vi "DropDetectionForLinkamForMultipleImages.vi"(6 "Circle Descriptor":cluster{"Min Radius":dbl, "Max Radius":dbl}={"Min Radius"=3.0, "Max Radius"=500.0}, 8 "error in":errorcluster, 9 "Image in":T2(plugin-control), 10 "Minimum match score":dbl=950.0) -> (0 "error out":errorcluster, 1 "Number of matches":i32, 2 "Matches (pixel)":T1(array[cluster]), 3 "Image Out":T2(plugin-control), 4 "Circles (Calibrated)":T3(array[cluster]) {"Position"."Y" format="%.2f"; "Position"."X" format="%.2f"})   [LabVIEW 2013]
uses:
  <vilib>/vision/NI_Vision_Development_Module.lvlib
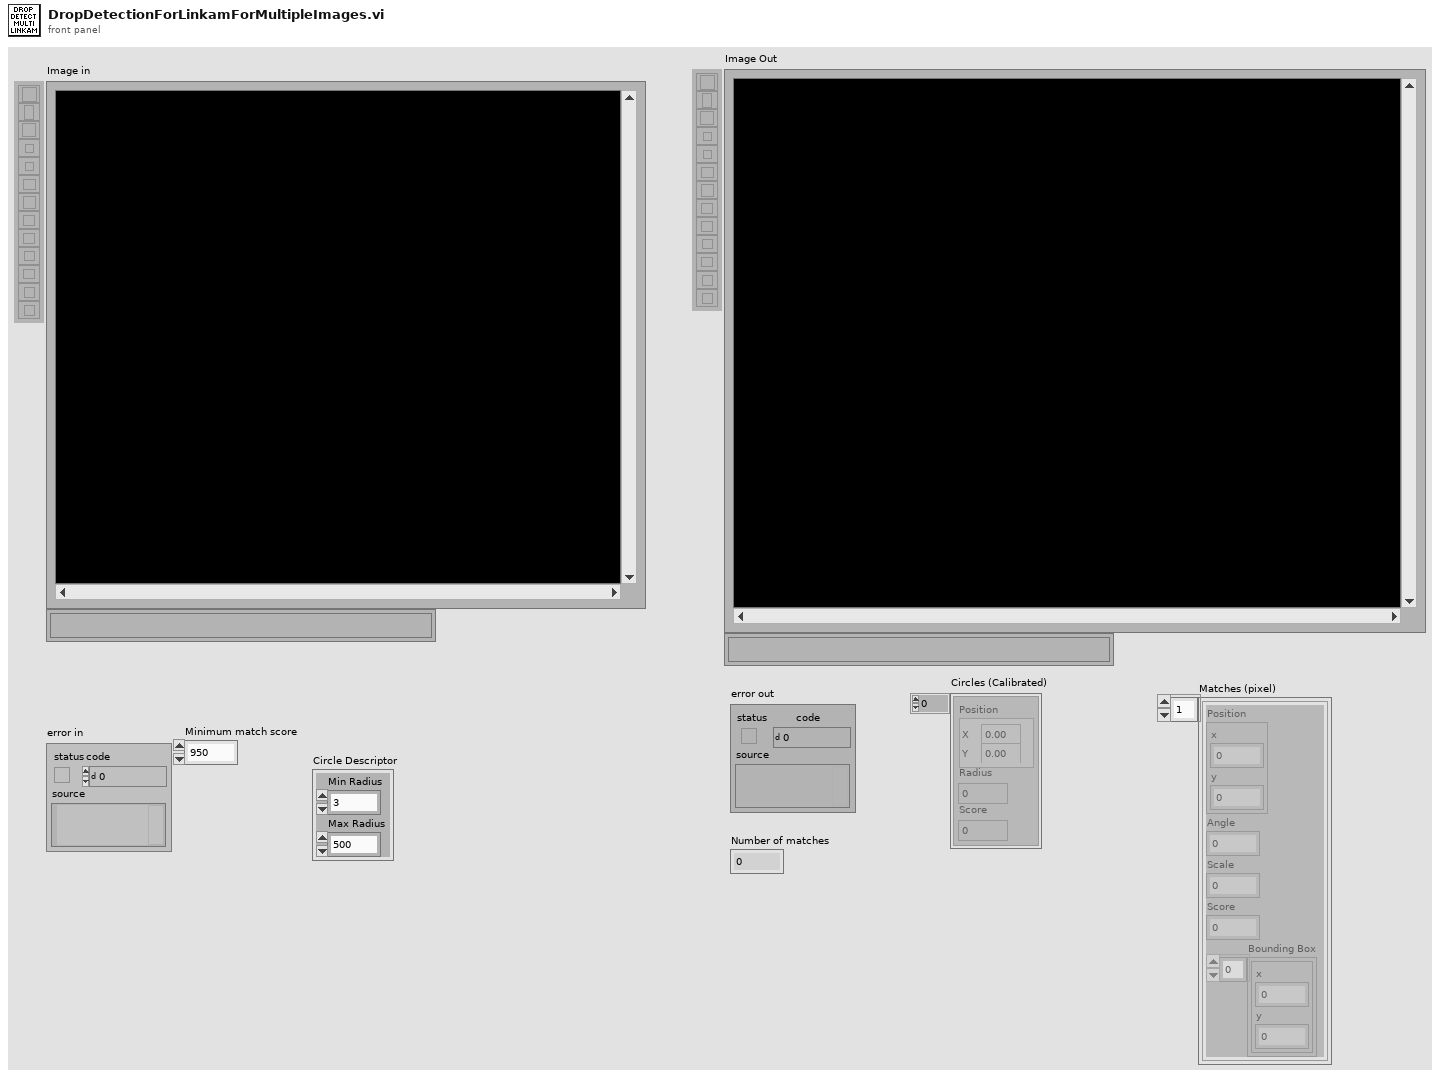
[diagram p1: front panel]
types:
  T1 = cluster{"Position":cluster{"x":sgl, "y":sgl}, "Angle":sgl, "Scale":sgl, "Score":sgl, "Bounding Box":cluster{"x":sgl, "y":sgl}[]}[]
  T2 = typedef "IMAQ Image.ctl" = refnum<image>
  T3 = cluster{"Position":cluster{"X":sgl, "Y":sgl}, "Radius":dbl, "Score":dbl}[]
  T4 = cluster{"Extraction Mode":u32, "Edge Threshold":i32, "Edge Filter Size":u32, "Min Length":i32, "Row Search Step Size":i32, "Col Search Step Size":i32, "Max Endpoint Gap":i32, "Closed":bool, "Subpixel":bool}
  T5 = cluster{"Rotation":bool, "Scale":bool, "Occlusion":bool, "Range Settings":cluster{"Match Constraints":u32, "Min":dbl, "Max":dbl}[]}
  T6 = cluster{"Global Rectangle":i32[], "Contours":cluster{"ID":enum32{"External", "Internal"}, "Type":u32, "Coordinates":i32[]}[]}
  T7 = cluster{"Position":cluster{"x":sgl, "y":sgl}, "Angle":sgl, "Scale":sgl, "Score":sgl, "Bounding Box":cluster{"x":sgl, "y":sgl}[]}
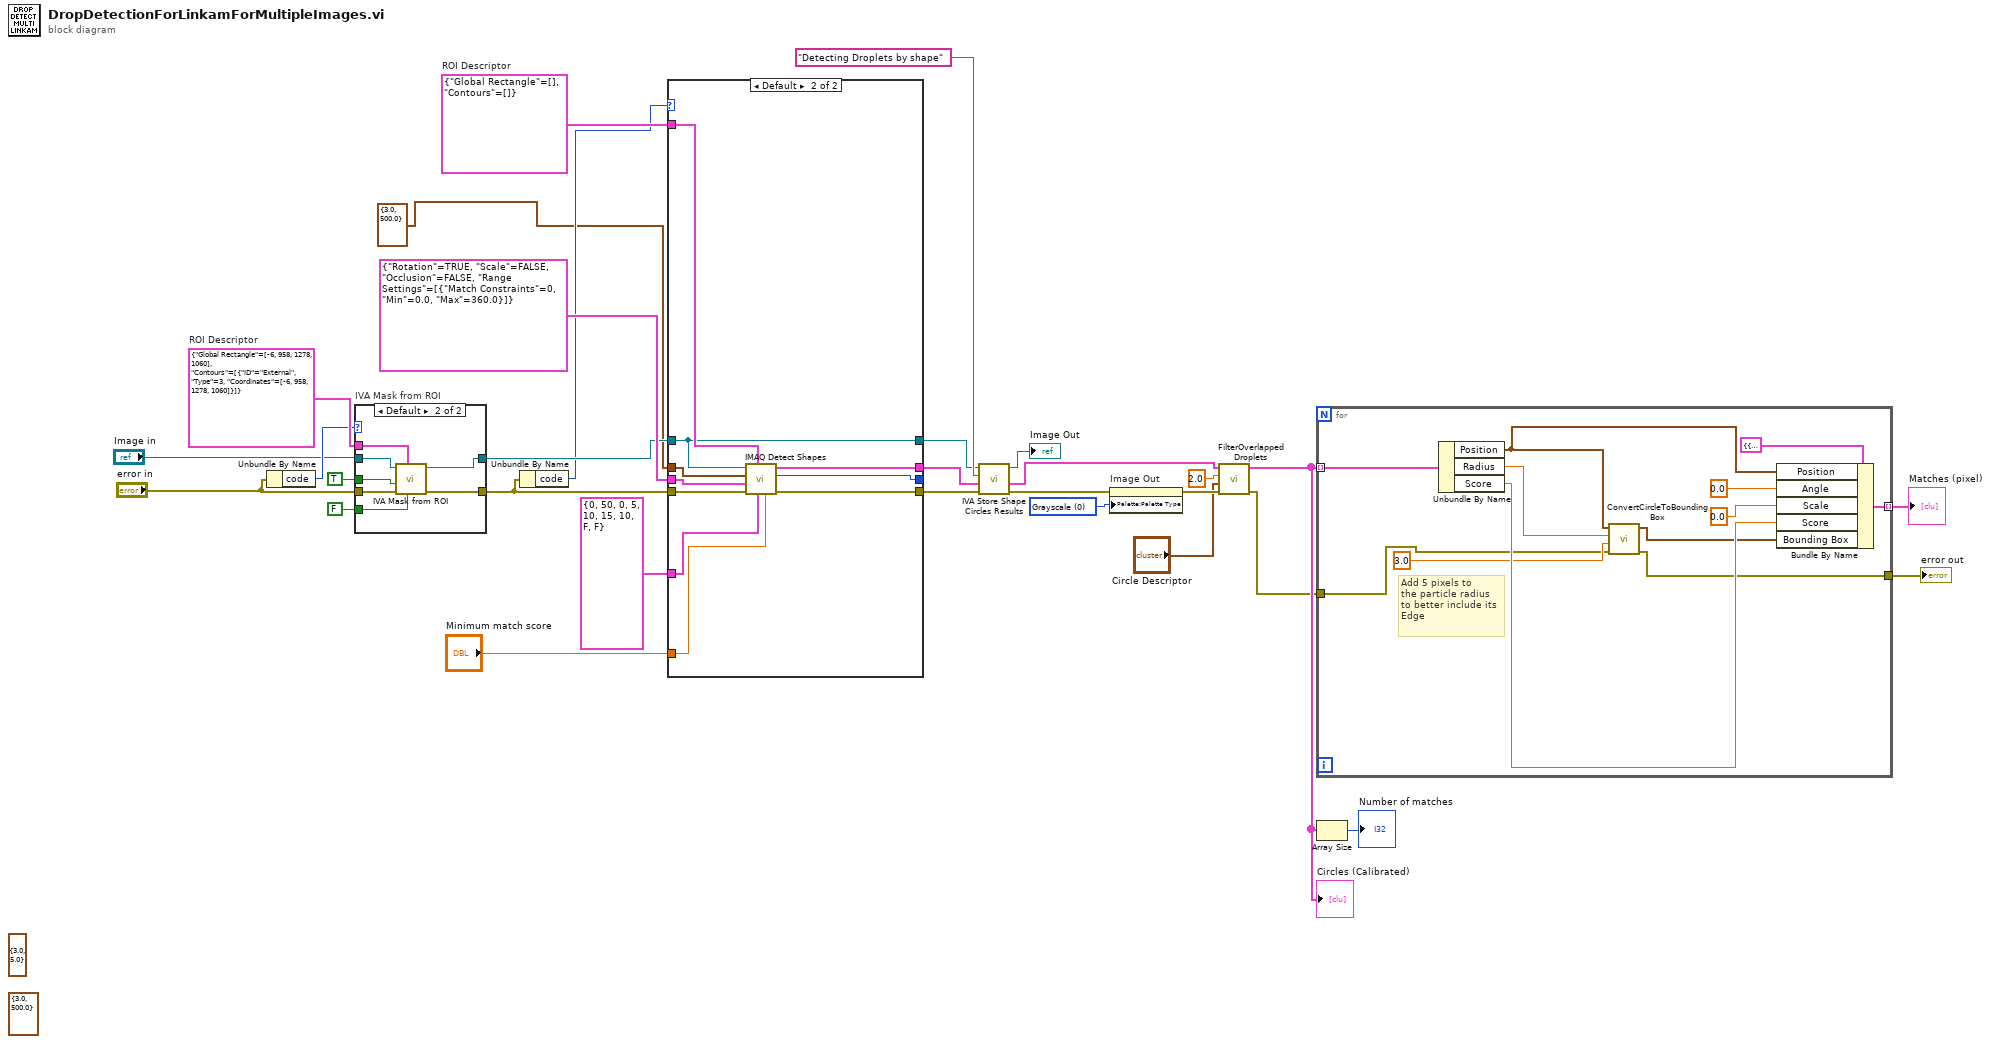
[diagram p0: block diagram]
diagram:
  (unwired) cluster{"Min Radius":dbl, "Max Radius":dbl} {"Min Radius"=3.0, "Max Radius"=500.0} ("Circle Descriptor")
  (unwired) cluster{"Min Radius":dbl, "Max Radius":dbl} {"Min Radius"=3.0, "Max Radius"=5.0} ("Circle Descriptor")
  w15 = u32 0 items=["Grayscale", "Binary", "Gradient", "Rainbow", "Temperature", "User Defined"] ("Palette")
  w24 = T6 {"Global Rectangle"=[], "Contours"=[]}  # ROI Descriptor
  w30 = T6 {"Global Rectangle"=[-6, 958, 1278, 1060], "Contours"=[{"ID"=enum."External", "Type"=3, "Coordinates"=[-6, 958, 1278, 1060]}]}  # ROI Descriptor
  n1 = Unbundle By Name("error in") -> ("code"=w27:i32)
  n2 = case "IVA Mask from ROI" shown="Default" w27 {
    tunnel: w30 -> [_ w38]
    tunnel: FALSE ("Shrink") -> [_ w37]
    tunnel: "Image in" -> [w31 w36]
    tunnel: "error in" -> [_ w35]
    tunnel: [_ w34] -> w19
    tunnel: [w31 w33] -> w22
    tunnel: TRUE ("Out / In") -> [_ w32]
    frame -1074396199, -1074396198 {
      # "Discard\nCoordinate\nSystem\nError"
    }
    frame Default {
      n3 = call <vilib>:"IVA Mask from ROI.vi"("Shrink"=w37, "ROI Descriptor"=w38, "error in (no error)"=w35, "Out / In"=w32, "Image Src"=w36) -> ("error out"=w34:errorcluster, "Image Out"=w33:T2)  [unwired: 5 out]
    }
  }
  n4 = Unbundle By Name(w19) -> ("code"=w18:i32)
  n5 = case shown="Default" w18 {
    tunnel: w19 -> [_ w49]
    tunnel: [_ w48] -> _
    tunnel: T5 {"Rotation"=TRUE, "Scale"=FALSE, "Occlusion"=FALSE, "Range Settings"=[{"Match Constraints"=0, "Min"=0.0, "Max"=360.0}]} ("Match Options") -> [_ w47]
    tunnel: T4 {"Extraction Mode"=0, "Edge Threshold"=50, "Edge Filter Size"=0, "Min Length"=5, "Row Search Step Size"=10, "Col Search Step Size"=15, "Max Endpoint Gap"=10, "Closed"=FALSE, "Subpixel"=FALSE} ("Curve Parameters") -> [_ w46]
    tunnel: "Minimum match score" -> [_ w45]
    tunnel: cluster{"Min Radius":dbl, "Max Radius":dbl} {"Min Radius"=3.0, "Max Radius"=500.0} ("Circle Descriptor") -> [_ w44]
    tunnel: w24 -> [_ w43]
    tunnel: [_ w42] -> w23
    tunnel: w22 -> [w39 w40]
    tunnel: [_ w41] -> w21
    tunnel: [w39 w40] -> w17
    frame -1074396199, -1074396198 {
      # "Discard Coordinate\nSystem Error"
    }
    frame Default {
      n6 = call-poly "IMAQ Detect Shapes"("Minimum match score"=w45, "Curve Parameters"=w46, "ROI Descriptor"=w43, "error in (no error)"=w49, "Match Options"=w47, "Circle Descriptor"=w44, "Image"=w40) -> ("error out"=w41:errorcluster, "Number of Matches Returned"=w48:i32, "Circles"=w42:T3)  [unwired: 2 out]
    }
  }
  n7 = call <vilib>:"IVA Store Shape Circles Results.vi"("error in (no error)"=w21, "Circles"=w23, "Step Name"="Detecting Droplets by shape", "Image in"=w17) -> ("error out"=w14:errorcluster, "Circles (Calibrated)"=w10:T3, "Image dup"=→"Image Out":T2)  [unwired: 5 out]
  n8 = property on="Image Out" class="ImageControl"(error in=w14, "Palette:Palette Type"=w15) -> (error out=w7:errorcluster)  [unwired: 1 in, 1 out]
  n9 = call "FilterOverlappedDroplets.vi"("error in (no error)"=w7, "Circle Descriptor"="Circle Descriptor", "Threshold (pixels)"=2.0, "Circles (Calibrated)"=w10) -> ("error out"=w4:errorcluster, "Circles (Calibrated) 2"=w8:T3)  [unwired: 6 in]
  "Circles (Calibrated)" <- w8
  n10 = for {
    tunnel: w8 -> [w60] mode=indexing
    tunnel: [w56] -> w11 mode=indexing
    tunnel: w4 -> [w51]
    tunnel: [w50] -> w3
    # "Add 5 pixels to\nthe particle radius \nto better include its\nEdge"
    n11 = Unbundle By Name(w60) -> ("Position"=w54:cluster{"X":sgl, "Y":sgl}, "Radius"=w53:dbl, "Score"=w59:dbl)
    n12 = call "ConvertCircleToBoundingBox.vi"("error in (no error)"=w51, "InflateBoxbyPixelNo"=3.0 ("y"), "Radius"=w53, "Position"=w54) -> ("error out"=w50:errorcluster, "Bounding Box"=w55:cluster{"x":sgl, "y":sgl}[])  [unwired: 6 in]
    n13 = Bundle By Name(cluster=T7 {"Position"={"x"=0.0, "y"=0.0}, "Angle"=0.0, "Scale"=0.0, "Score"=0.0, "Bounding Box"=[]} ("element"), "Position"=w54, "Angle"=sgl 0.0, "Scale"=sgl 0.0, "Score"=w59, "Bounding Box"=w55) -> (w56:T7)
  }
  "error out" <- w3
  "Matches (pixel)" <- w11
  n14 = Array Size(array=w8) -> (size(s)=→"Number of matches":i32)
